vi "Launch.vi"(9 "Queue Actor":refnum<class "Queue Actor.lvclass">, 10 "Event Actor":refnum<class "Event Actor.lvclass">) -> (0 "error out":errorcluster, 2 "Event Actor":refnum<class "Event Actor.lvclass">)   [LabVIEW 2021, in "Event Actor.lvclass"]
uses:
  Event Actor.lvclass
  Queue Actor/Queue Actor.lvclass
  Loop Wrapper.vi
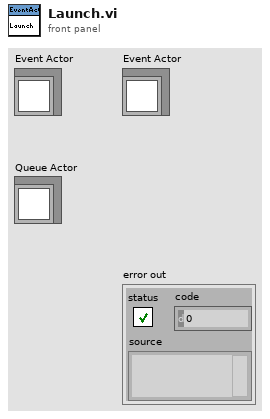
[diagram p1: front panel]
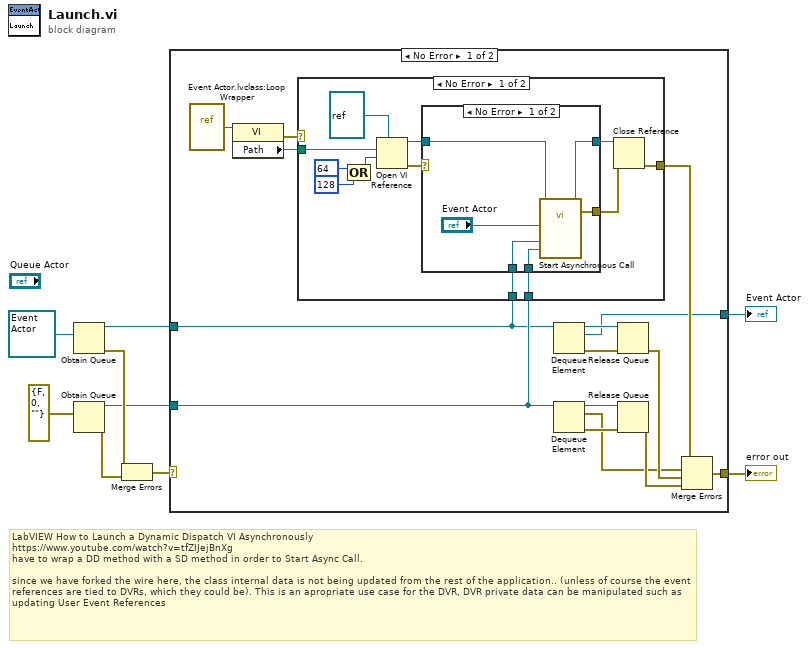
[diagram p0: block diagram]
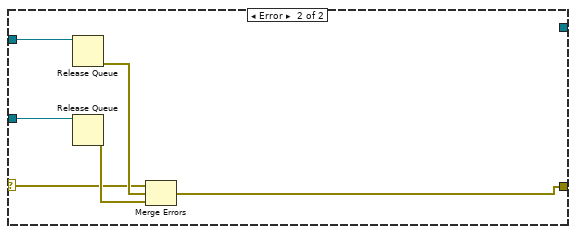
[diagram p4: hidden frame]
diagram:
  # "LabVIEW How to Launch a Dynamic Dispatch VI Asynchronously\nhttps://www.youtube.com/watch?v=tfZIJejBnXg\nhave to wrap a DD method with a SD method in order to Start Async Call.\n\nsince we have forked the wire here, the class internal data is not being updated from the rest of the application.. (unless of course the event references are tied to DVRs, which they could be). This is an apropriate use case for the DVR, DVR private data can be manipulated such as updating User Event References"
  n1 = Obtain Queue(element data type=refnum<class "Event Actor.lvclass"> refnum ("Helper Loop.lvclass")) -> (queue out=w6:refnum<queue>, error out=w5:errorcluster)  [unwired: 4 in, 1 out]
  n2 = Obtain Queue(element data type=errorcluster {"status"=FALSE, "code"=0, "source"=""} ("error out")) -> (queue out=w1:refnum<queue>, error out=w2:errorcluster)  [unwired: 4 in, 1 out]
  n3 = Merge Errors(w5, w2) -> (w3:errorcluster)
  n4 = case shown="No Error" w3 {
    selector: w3 -> [_ w46]
    tunnel: [w10 _] -> w9
    tunnel: [w20 w50] -> w8
    tunnel: w6 -> [w11 w51]
    tunnel: w1 -> [w18 w48]
    frame No Error {
      n5 = vi-ref "Event Actor.lvclass:Loop Wrapper.vi"() -> (w22:refnum<vi>)
      n6 = property class="VI"(reference=w22) -> (error out=w23:errorcluster, "Path"=w21:path)  [unwired: 1 in, 1 out]
      n7 = case shown="No Error" w23 {
        selector: w23 -> [_ w45]
        tunnel: [w34 w45] -> w24
        tunnel: w21 -> [w27 _]
        tunnel: w11 -> [w26 _]
        tunnel: w18 -> [w25 _]
        frame No Error {
          n8 = Compound Arithmetic op=OR(64 ("options: Multiple Clones,\n  Fire & Forget"), 128 ("options: Multiple Clones,\n  Fire & Forget")) -> (w32:i32)
          n9 = Open VI Reference(type specifier VI Refnum (for type only)=refnum<vi> refnum, vi path=w27, options=w32) -> (vi reference=w29:refnum<vi>, error out=w30:errorcluster)  [unwired: 3 in]
          n10 = case shown="No Error" w30 {
            selector: w30 -> [_ w44]
            tunnel: [w41 w43] -> w36
            tunnel: [w40 w44] -> w35
            tunnel: w29 -> [w42 w43]
            tunnel: w26 -> [w39 _]
            tunnel: w25 -> [w38 _]
            frame No Error {
              n11 = call-by-ref "Start Asynchronous Call"(reference=w42, "Error Queue"=w38, "Helper Loop Queue"=w39, "Helper Loop in"="Event Actor") -> (reference out=w41:refnum<vi>, error out=w40:errorcluster)  [unwired: 10 in]
            }
            frame Error {
            }
          }
          n12 = Close Reference(reference=w36, error in (no error)=w35) -> (error out=w34:errorcluster)
        }
        frame Error {
        }
      }
      n13 = Dequeue Element(queue=w11) -> (queue out=w19:refnum<queue>, element=w10:refnum<class "Event Actor.lvclass">, error out=w16:errorcluster)  [unwired: 2 in, 1 out]
      n14 = Dequeue Element(queue=w18) -> (queue out=w17:refnum<queue>, element=w12:errorcluster, error out=w14:errorcluster)  [unwired: 2 in, 1 out]
      n15 = Release Queue(queue=w19, error in (no error)=w16) -> (error out=w15:errorcluster)  [unwired: 1 in, 2 out]
      n16 = Release Queue(queue=w17, error in (no error)=w14) -> (error out=w13:errorcluster)  [unwired: 1 in, 2 out]
      n17 = Merge Errors(w24, w12, w15, w13) -> (w20:errorcluster)
    }
    frame Error {
      n18 = Release Queue(queue=w51) -> (error out=w49:errorcluster)  [unwired: 2 in, 2 out]
      n19 = Release Queue(queue=w48) -> (error out=w47:errorcluster)  [unwired: 2 in, 2 out]
      n20 = Merge Errors(w46, w49, w47) -> (w50:errorcluster)
    }
  }
  "error out" <- w8
  "Event Actor" <- w9
